vi "Translation2d_Div.vi"(9 "Scalar":dbl, 11 "In Translation":T1 {"Y" format="%14.3f"; "X" format="%14.3f"}) -> (3 "Out Translation":T1 {"Y" format="%14.3f"; "X" format="%14.3f"})   [LabVIEW 2019, in "Trajectory_Library.lvlib"]
doc: "Divides the translation by a scalar and returns the new translation.\n\nParameters:\n - In Translation - This translation data structure\n - scalar - The value to divide the translation by\n\nResult:\n - Out Translation - The resulting translation"
uses:
  Trajectory_Library.lvlib
  TypeDef/TRANSLATION2D.ctl
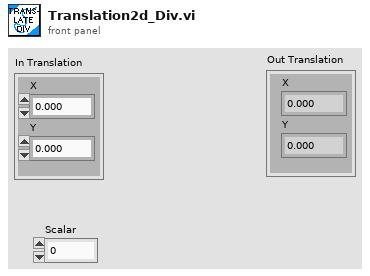
[diagram p1: front panel]
types:
  T1 = typedef "Trajectory_Library.lvlib/TRANSLATION2D.ctl" = cluster{"X":dbl, "Y":dbl}
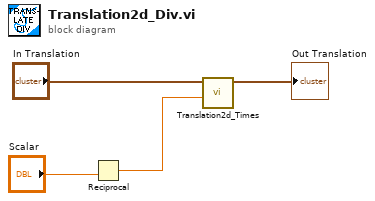
[diagram p0: block diagram]
diagram:
  n1 = Reciprocal(x="Scalar") -> (1/x=w1:dbl)
  n2 = call "Translation2d_Times.vi"("Scalar"=w1, "In Translation"="In Translation") -> ("Out Translation"=→"Out Translation":T1)  [unwired: 9 in]
